vi "PhotocellQ2.vi"() -> ()   [LabVIEW 2021, in "LabVIEW Interface for Arduino.lvlib"]
doc: "An example that uses the Arduino to read the value of a photocell."
uses:
  <vilib>/LabVIEW Interface for Arduino/LabVIEW Interface for Arduino.lvlib
  <vilib>/LabVIEW Interface for Arduino/Type Defs/Analog Pin.ctl
panel:
  out "Boolean 6":bool
  out "Boolean 5":bool
  out "Boolean 4":bool
  out "Boolean 3":bool
  out "Boolean 2":bool
  out "Boolean":bool
  in  "VISA resource":refnum<visa-resource-name>
  in  "Stop":bool
  out "Light Intensity (0 - 100)":dbl(knob) scale=0.0..100.0
  in  "Photo Cell Pin (AI 0-5)":T1=enum."Anlog In 1"
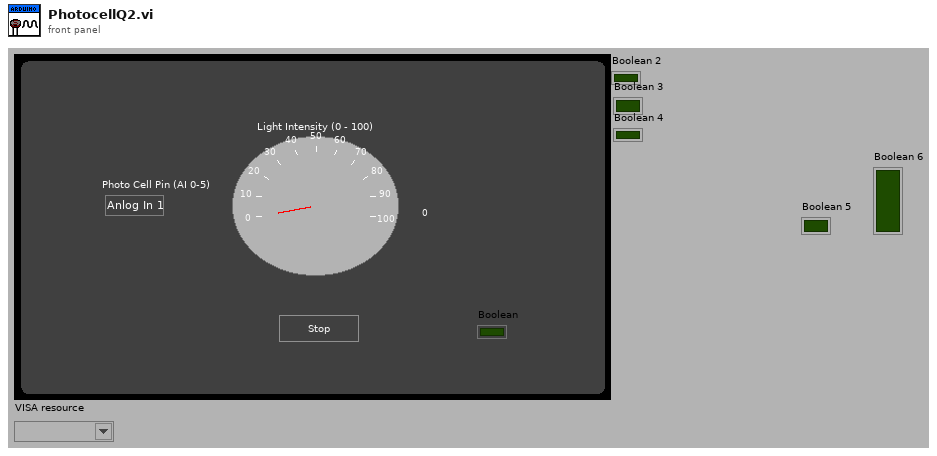
[diagram p1: front panel]
types:
  T1 = typedef "LabVIEW Interface for Arduino.lvlib/Analog Pin.ctl" = enum8{"Anlog In 0", "Anlog In 1", "Anlog In 2", "Anlog In 3", "Anlog In 4", "Anlog In 5"}
  T2 = typedef "LabVIEW Interface for Arduino.lvlib/Arduino Resource.ctl" = cluster{"VISA resource":refnum<visa-resource-name>, "Board Type":T3, "Connection Type":enum8{"USB / Serial"}, "Bytes Per Packet (15)":u8}
  T3 = typedef "LabVIEW Interface for Arduino.lvlib/Board Type.ctl" = enum16{"Uno", "Dimuelanove w/Atmega 328", "Mega 2560"}
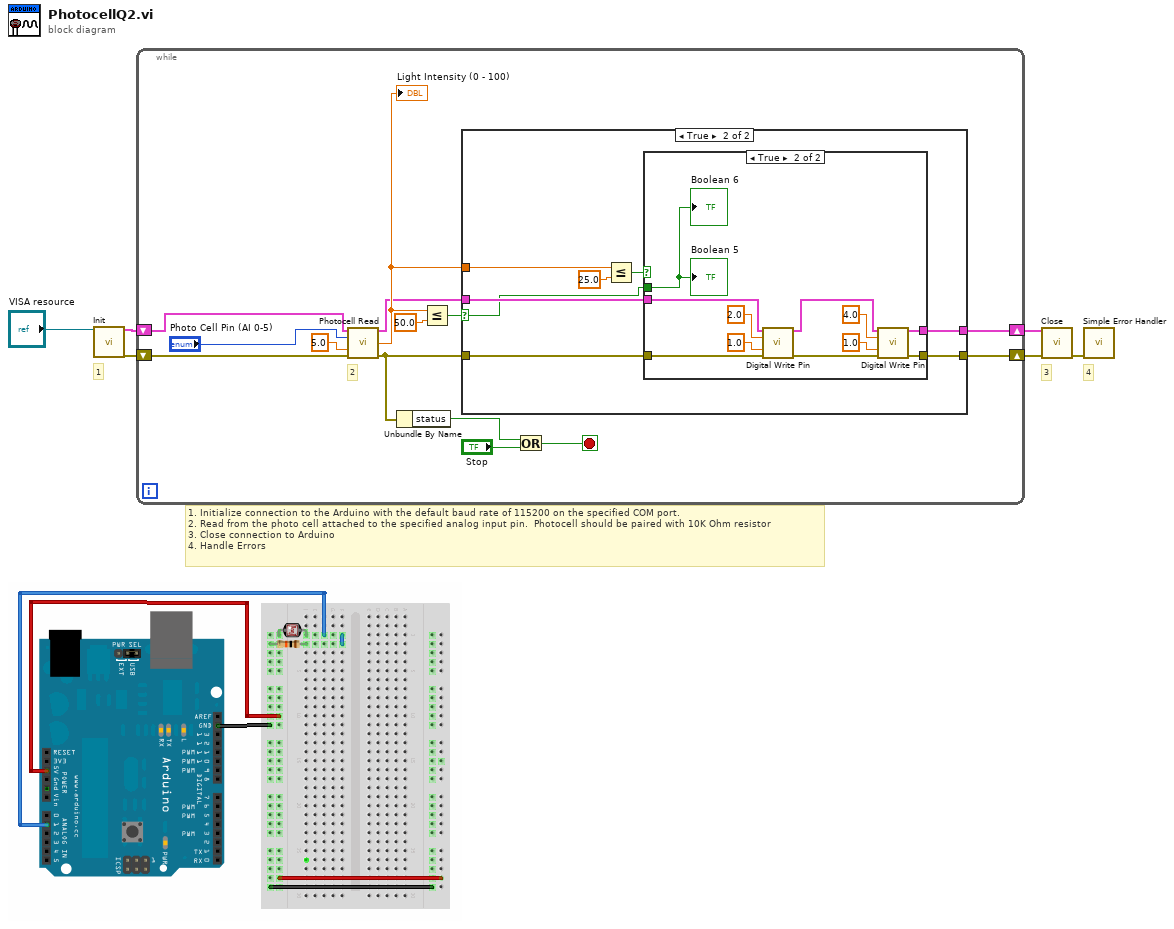
[diagram p0: block diagram]
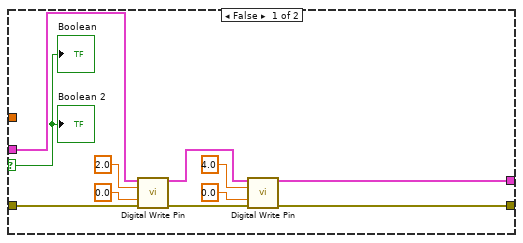
[diagram p2: hidden frame]
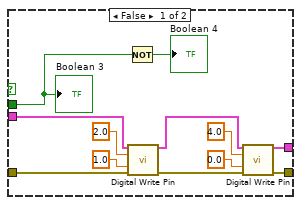
[diagram p3: hidden frame]
diagram:
  # "1. Initialize connection to the Arduino with the default baud rate of 115200 on the specified COM port.\n2. Read from the photo cell attached to the specified analog input pin.  Photocell should be paired with 10K Ohm resistor\n3. Close connection to Arduino\n4. Handle Errors"
  # "4"
  # "3"
  # "1"
  n1 = call <vilib>:"Init.vi"("VISA resource"="VISA resource") -> ("Arduino Resource"=w5:T2, "error out"=w4:errorcluster)  [unwired: 17 in]
  n2 = while {
    shift-right: [w7] -> w6
    shift-left: w4 -> [w20]
    shift-right: [w8] -> w2
    shift-left: w5 -> [w14]
    stop <- w15 stop-if-true
    # "2"
    n3 = call <vilib>:"Photocell Read.vi"("Arduino Resource"=w14, "Photo Cell Pin (0)"="Photo Cell Pin (AI 0-5)", "Vcc (5)"=5.0 ("Vcc"), "error in"=w20) -> ("Arduino Resource"=w10:T2, "Light Intensity (0 - 100)"=w11:dbl, "error out"=w9:errorcluster)  [unwired: 9 in]
    "Light Intensity (0 - 100)" <- w11
    n4 = Unbundle By Name(w9) -> ("status"=w17:bool)
    n5 = Less Or Equal?(x=w11, y=50.0) -> (x <= y?=w12:bool)
    n6 = case shown="True" w12 {
      selector: w12 -> [w21 w32]
      tunnel: w11 -> [_ w39]
      tunnel: w10 -> [w25 w36]
      tunnel: w9 -> [w24 w35]
      tunnel: [w22 w34] -> w8
      tunnel: [w23 w33] -> w7
      frame False {
        n7 = call <vilib>:"Digital Write Pin.vi"("Arduino Resource"=w25, "Digital I/O Pin (0)"=2.0, "Value (0)"=0.0, "error in"=w24) -> ("Arduino Resource"=w27:T2, "error out"=w26:errorcluster)  [unwired: 10 in]
        n8 = call <vilib>:"Digital Write Pin.vi"("Arduino Resource"=w27, "Digital I/O Pin (0)"=4.0, "Value (0)"=0.0, "error in"=w26) -> ("Arduino Resource"=w22:T2, "error out"=w23:errorcluster)  [unwired: 10 in]
        "Boolean" <- w21
        "Boolean 2" <- w21
      }
      frame True {
        n9 = Less Or Equal?(x=w39, y=25.0) -> (x <= y?=w37:bool)
        n10 = case shown="True" w37 {
          tunnel: w36 -> [w45 w57]
          tunnel: w35 -> [w44 w58]
          tunnel: [w42 w55] -> w34
          tunnel: [w43 w53] -> w33
          tunnel: w32 -> [w40 w52]
          frame False {
            n11 = Not(x=w40) -> (.not. x?=→"Boolean 4":bool)
            n12 = call <vilib>:"Digital Write Pin.vi"("Arduino Resource"=w45, "Digital I/O Pin (0)"=2.0, "Value (0)"=1.0, "error in"=w44) -> ("Arduino Resource"=w47:T2, "error out"=w46:errorcluster)  [unwired: 10 in]
            n13 = call <vilib>:"Digital Write Pin.vi"("Arduino Resource"=w47, "Digital I/O Pin (0)"=4.0, "Value (0)"=0.0, "error in"=w46) -> ("Arduino Resource"=w42:T2, "error out"=w43:errorcluster)  [unwired: 10 in]
            "Boolean 3" <- w40
          }
          frame True {
            n14 = call <vilib>:"Digital Write Pin.vi"("Arduino Resource"=w57, "Digital I/O Pin (0)"=2.0, "Value (0)"=1.0, "error in"=w58) -> ("Arduino Resource"=w56:T2, "error out"=w54:errorcluster)  [unwired: 10 in]
            n15 = call <vilib>:"Digital Write Pin.vi"("Arduino Resource"=w56, "Digital I/O Pin (0)"=4.0, "Value (0)"=1.0, "error in"=w54) -> ("Arduino Resource"=w55:T2, "error out"=w53:errorcluster)  [unwired: 10 in]
            "Boolean 5" <- w52
            "Boolean 6" <- w52
          }
        }
      }
    }
    n16 = Or(x=w17, y="Stop") -> (x .or. y?=w15:bool)
  }
  n17 = call <vilib>:"Close.vi"("Arduino Resource"=w2, "error in"=w6) -> ("error out"=w3:errorcluster)  [unwired: 13 in]
  n18 = call <vilib>:"Simple Error Handler.vi"("error in (no error)"=w3) -> ()  [unwired: 4 in, 5 out]
